vi "Bundle Script_Select Constant Class.vi"(8 "error in":errorcluster, 10 "ID String":string, 11 "Affected Items":T1) -> (0 "error out":errorcluster, 2 "Objects":refnum<vi>[](array[refnum]))   [LabVIEW 2023]
uses:
  top/BundleMagic.ctl
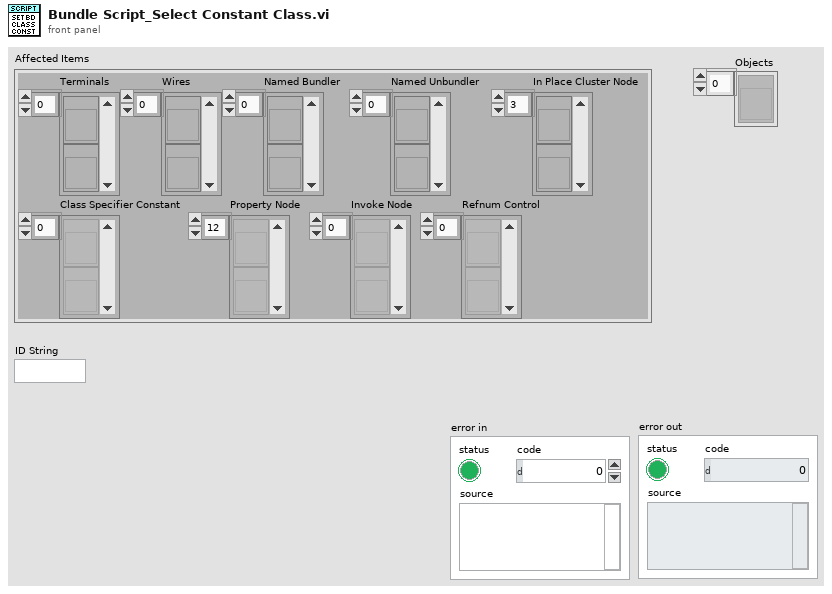
[diagram p1: front panel]
types:
  T1 = typedef "BundleMagic.ctl" = cluster{"Terminals":refnum<vi>[], "Wires":refnum<vi>[], "Named Bundler":refnum<vi>[], "Named Unbundler":refnum<vi>[], "In Place Cluster Node":refnum<vi>[], "Class Specifier Constant":refnum<vi>[], "Property Node":refnum<vi>[], "Invoke Node":refnum<vi>[], "Refnum Control":refnum<vi>[]}
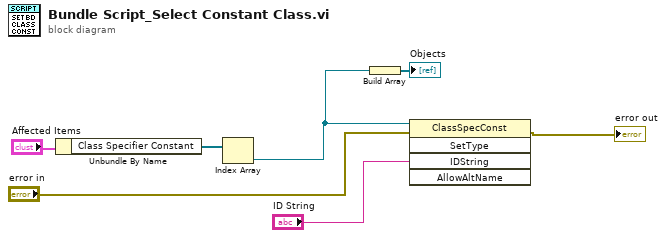
[diagram p0: block diagram]
diagram:
  n1 = Unbundle By Name("Affected Items") -> ("Class Specifier Constant"=w6:refnum<vi>[])
  n2 = Index Array(array=w6) -> (element=w2:refnum<vi>)  [unwired: 1 in]
  n3 = Build Array(w2) -> (→"Objects":refnum<vi>[])
  n4 = invoke class="ClassSpecConst" method="SetType"(reference=w2, error in="error in", "IDString"="ID String") -> (error out=→"error out":errorcluster)  [unwired: 2 in, 4 out]
